vi "Start Measurement.vi"(8 "error in (no error)":errorcluster, 11 "Keithley2400 in":refnum<class "Keithley2400.lvclass">) -> (0 "error out":errorcluster, 3 "Keithley2400 out":refnum<class "Keithley2400.lvclass">)   [LabVIEW 2015, in "Keithley2400.lvclass"]
uses:
  Keithley2400.lvclass
  Meter/Keithley Meter Parameters.ctl
  Meter/KeithleyMeter Function.ctl
  Instrument/Read VISA Resource.vi
  OO Devices/Device/Read Controls Snapshot.vi
  Instrument/Write VISA Resource.vi
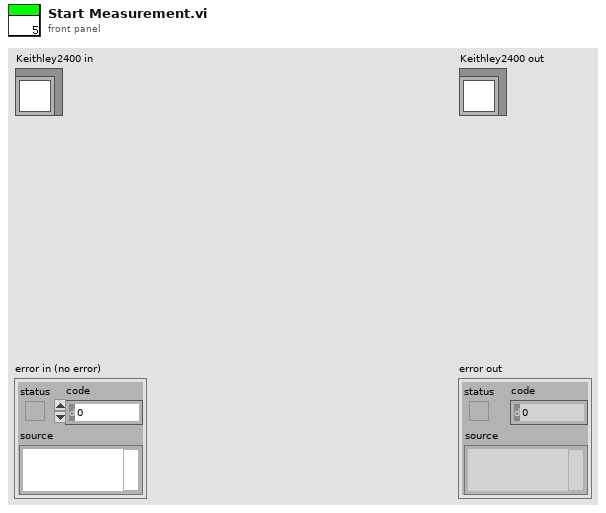
[diagram p1: front panel]
types:
  T1 = typedef "Keithley Meter Parameters.ctl" = cluster{"Range (-1: auto)":dbl, "Integration Time (NPLCs)":dbl, "Function":T2, "W Offset comp":bool, "4-wire W":bool, "Scale":dbl, "Offset":dbl}
  T2 = typedef "KeithleyMeter Function.ctl" = enum16{"VOLTAGE", "CURRENT", "RESISTANCE"}
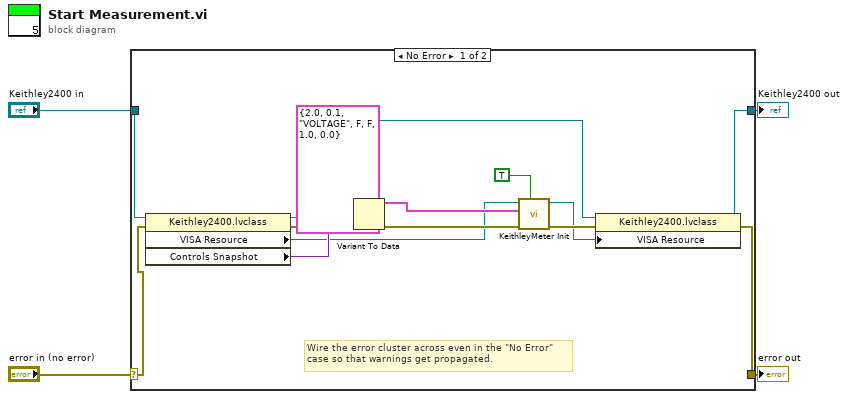
[diagram p0: block diagram]
diagram:
  n1 = case shown="No Error" "error in (no error)" {
    selector: "error in (no error)" -> [w7 w20]
    tunnel: [w6 w20] -> w3
    tunnel: [w8 w19] -> w1
    tunnel: "Keithley2400 in" -> [w9 w19]
    frame No Error {
      # "Wire the error cluster across even in the \"No Error\"\ncase so that warnings get propagated."
      n2 = property class="Keithley2400.lvclass"(reference=w9, error in=w7) -> (reference out=w17:refnum<class "Keithley2400.lvclass">, error out=w12:errorcluster, "VISA Resource"=w11:refnum<visa-resource-name>, "Controls Snapshot"=w13:variant)
      n3 = Variant To Data(error in=w12, type=T1 {"Range (-1: auto)"=2.0, "Integration Time (NPLCs)"=0.1, "Function"=enum."VOLTAGE", "W Offset comp"=FALSE, "4-wire W"=FALSE, "Scale"=1.0, "Offset"=0.0} ("Parameters"), Variant=w13) -> (data=w18:T1, error out=w15:errorcluster)
      n4 = call "KeithleyMeter Init.vi"("Source-meter"=TRUE ("Set Elements"), "Error In"=w15, "Parameters"=w18, "VISA resource name"=w11) -> ("Error Out"=w16:errorcluster, "VISA resource name out"=w10:refnum<visa-resource-name>)  [unwired: 6 in]
      n5 = property class="Keithley2400.lvclass"(reference=w17, error in=w16, "VISA Resource"=w10) -> (reference out=w8:refnum<class "Keithley2400.lvclass">, error out=w6:errorcluster)
    }
    frame Error {
    }
  }
  "error out" <- w3
  "Keithley2400 out" <- w1
